vi "Voice Status.vi"(3 "error in (no error)":errorcluster, 5 "SpeechLib.ISpeechVoice (In)":refnum<k7>) -> (0 "error out":errorcluster, 1 "Status (T: Done)":bool, 2 "SpeechLib.ISpeechVoice (Out)":refnum<k7>)   [LabVIEW 2018]
doc: "This SubVI checks on the status of the voice and returns a 1 (TRUE) if the voice is done speaking the text or a 0 (FALSE) if the voice is in progress."
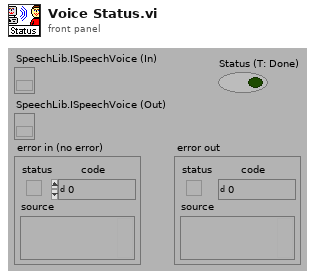
[diagram p1: front panel]
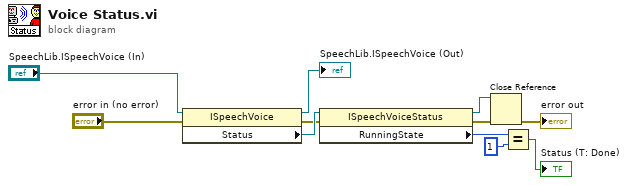
[diagram p0: block diagram]
diagram:
  n1 = property class="ISpeechVoice"(reference="SpeechLib.ISpeechVoice (In)", error in="error in (no error)") -> (reference out=→"SpeechLib.ISpeechVoice (Out)":refnum<k7>, error out=w3:errorcluster, "Status"=w8:refnum<k7>)
  n2 = property class="ISpeechVoiceStatus"(reference=w8, error in=w3) -> (reference out=w5:refnum<k7>, error out=w4:errorcluster, "RunningState"=w9:i32)
  n3 = Close Reference(reference=w5, error in (no error)=w4) -> (error out=→"error out":errorcluster)
  n4 = Equal?(x=w9, y=1) -> (x = y?=→"Status (T: Done)":bool)
